vi "setFrame.vi"(6 "Image Name":string="untitled", 8 "error in (no error)":errorcluster, 9 "Y Resolution":i32=1500, 10 "X Resolution":i32=1930, 11 "Stimulus in":refnum<class "Stimulus.lvclass">) -> (0 "error out":errorcluster, 3 "Stimulus out":refnum<class "Stimulus.lvclass">)   [LabVIEW 2013, in "Stimulus.lvclass"]
uses:
  Stimulus.lvclass
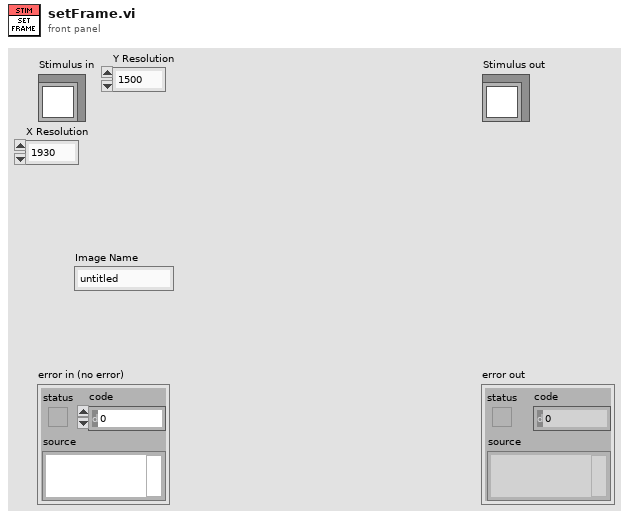
[diagram p1: front panel]
types:
  T1 = typedef "IMAQ Image.ctl" = refnum<image>
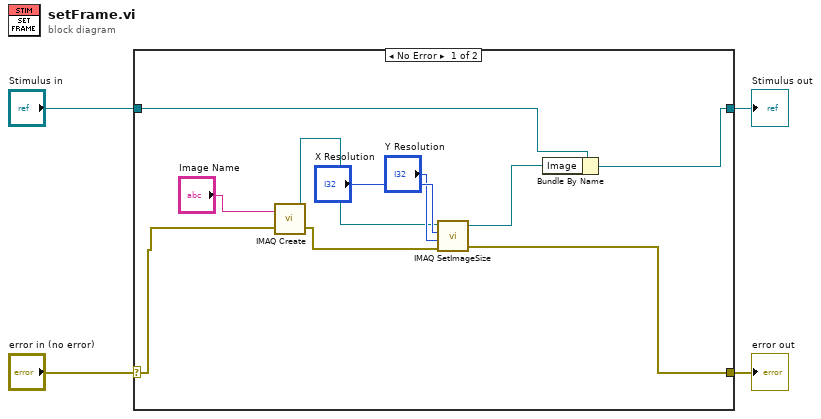
[diagram p0: block diagram]
diagram:
  n1 = case shown="No Error" "error in (no error)" {
    selector: "error in (no error)" -> [w5 w16]
    tunnel: [w9 w16] -> w3
    tunnel: [w11 w15] -> w1
    tunnel: "Stimulus in" -> [w12 w15]
    frame No Error {
      n2 = call "IMAQ Create"("Image Name"="Image Name", "error in (no error)"=w5) -> ("New Image"=w7:T1, "error out"=w6:errorcluster)  [unwired: 3 in]
      n3 = call "IMAQ SetImageSize"("error in (no error)"=w6, "Y Resolution"="Y Resolution", "X Resolution"="X Resolution", "Image"=w7) -> ("error out"=w9:errorcluster, "Image Out"=w10:T1)  [unwired: 1 in]
      n4 = Bundle By Name(cluster=w12, "Image"=w10) -> (w11:refnum<class "Stimulus.lvclass">)
    }
    frame Error {
    }
  }
  "error out" <- w3
  "Stimulus out" <- w1
